vi "calcbuffers.vi"(3 "size":i32) -> (0 "wfsize":i32, 1 "# of frames":i32)   [LabVIEW 2015]
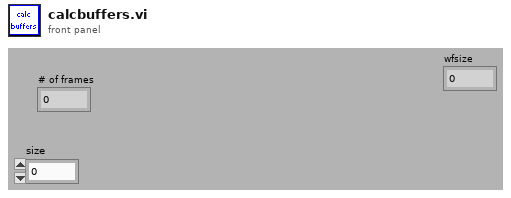
[diagram p1: front panel]
types:
  T1 = typedef "LVRectTypeDef.ctl" = cluster{"Left":i16, "Top":i16, "Right":i16, "Bottom":i16}
  T2 = cluster{"Xpixels":i32, "Vxminref":dbl, "Vxmaxref":dbl, "P":dbl, "Ypixels":i32, "Vyminref":dbl, "Vymaxref":dbl, "srate":sgl, "sAOxy":i32, "timeout":dbl, "type":string, "date":string, "time":string, "Colormap":u16, "Drawing Mode":u16, "Scanning Mode":u16, "square pixels":bool, "square matrix":bool, "Xpixels Img":i32, "Vx-min Img":dbl, "VX-max Img":dbl, "Ypixels Img":i32, "Vy-min Img":dbl, "Vy-max Img ":dbl, "Angle Img":dbl, "autoshutter":bool, "finite":bool, "cont":bool, "wavdet":bool, "measpoints":i32, "avpp":i32, "bufferAO":i32, "bufferAI":i32, "starttick":u32, "waveform":path, "Vx-ref":dbl, "Vy-ref":dbl, "refreshrate":dbl, "refreshbuffer":i32, "tt_cycles":i32, "motorref":refnum<k7>, "mirrorswitch":refnum<k7>, "sample mode":i32, "maxbufferAI":i32, "sampletreshold":dbl, "srateAODO":sgl, "bin":sgl, "Pel":sgl, "Angle draw":dbl, "srate Img":sgl, "ROIimg_plotbounds":T1, "auto OD":bool, "ODfilt":u16, "reset AO_DO":bool, "aAI":i32[], "aCI":i32[], "aAO":u32[], "aDO":u32[], "refwfsize":dbl}
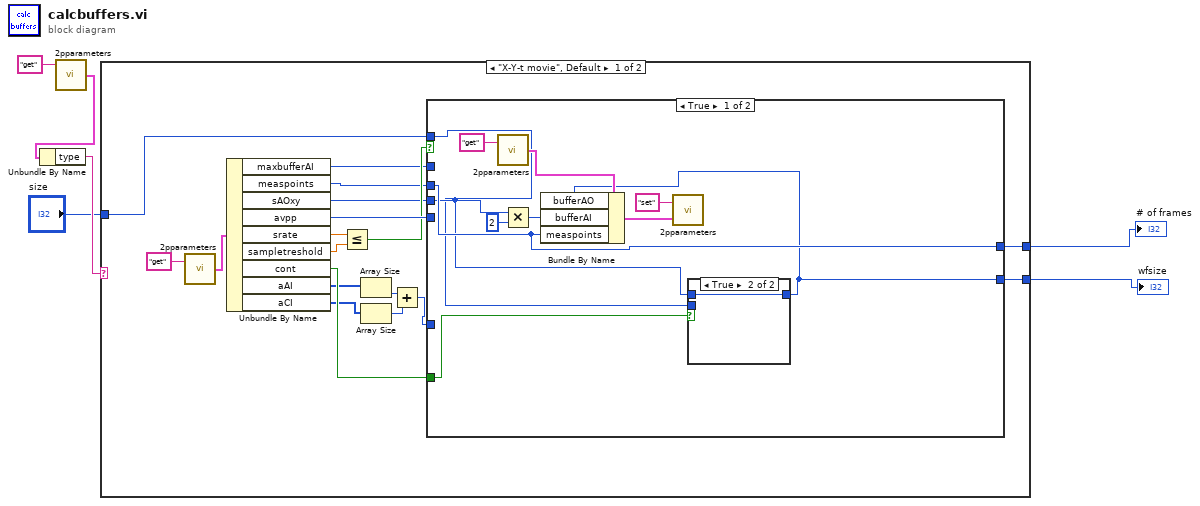
[diagram p0: block diagram]
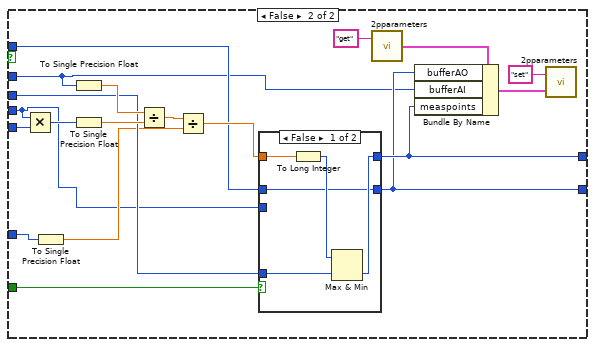
[diagram p3: hidden frame]
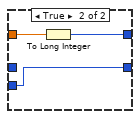
[diagram p4: hidden frame]
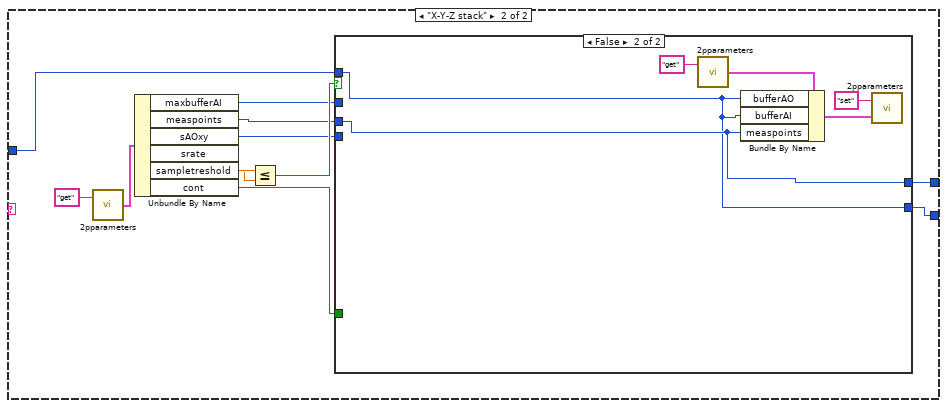
[diagram p5: hidden frame]
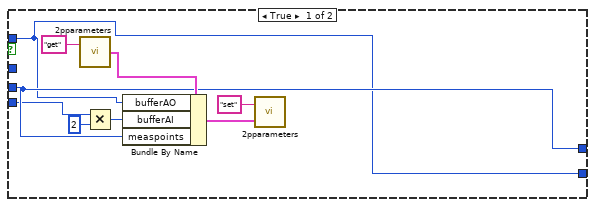
[diagram p6: hidden frame]
diagram:
  n1 = call "2pparameters.vi"("command"="get") -> ("params out"=w5:T2)  [unwired: 1 in]
  n2 = Unbundle By Name(w5) -> ("type"=w4:string)
  n3 = case shown="\"X-Y-t movie\", Default" w4 {
    tunnel: "size" -> [w9 w66]
    tunnel: [w8 w67] -> w2
    tunnel: [w7 w65] -> w1
    frame "X-Y-t movie", Default {
      n4 = call "2pparameters.vi"("command"="get") -> ("params out"=w23:T2)  [unwired: 1 in]
      n5 = Unbundle By Name(w23) -> ("maxbufferAI"=w16:i32, "measpoints"=w18:i32, "sAOxy"=w19:i32, "avpp"=w22:i32, "srate"=w21:sgl, "sampletreshold"=w17:dbl, "cont"=w15:bool, "aAI"=w14:i32[], "aCI"=w13:i32[])
      n6 = Less Or Equal?(x=w21, y=w17) -> (x <= y?=w20:bool)
      n7 = Array Size(array=w14) -> (size(s)=w12:i32)
      n8 = Array Size(array=w13) -> (size(s)=w11:i32)
      n9 = Add(x=w12, y=w11) -> (x+y=w10:i32)
      n10 = case shown="True" w20 {
        tunnel: w19 -> [w27 w40]
        tunnel: w22 -> [_ w52]
        tunnel: w10 -> [_ w47]
        tunnel: w18 -> [w29 w44]
        tunnel: w15 -> [w28 w45]
        tunnel: w16 -> [_ w38]
        tunnel: w9 -> [w26 w41]
        tunnel: [w29 w43] -> w8
        tunnel: [w25 w39] -> w7
        frame True {
          n11 = call "2pparameters.vi"("command"="get") -> ("params out"=w35:T2)  [unwired: 1 in]
          n12 = Multiply(x=w27, y=2) -> (x*y=w30:i32)
          n13 = case shown="True" w28 {
            tunnel: w27 -> [_ w37]
            tunnel: [w36 w37] -> w25
            tunnel: w26 -> [w36 _]
            frame False {
            }
            frame True {
            }
          }
          n14 = Bundle By Name(cluster=w35, "bufferAO"=w25, "bufferAI"=w30, "measpoints"=w29) -> (w34:T2)
          n15 = call "2pparameters.vi"("Params in"=w34, "command"="set") -> ()  [unwired: 1 out]
        }
        frame False {
          n16 = Multiply(x=w40, y=w52) -> (x*y=w51:i32)
          n17 = To Single Precision Float(number=w47) -> (single precision float=w42:sgl)
          n18 = To Single Precision Float(number=w38) -> (single precision float=w50:sgl)
          n19 = To Single Precision Float(number=w51) -> (single precision float=w49:sgl)
          n20 = Divide(x=w50, y=w49) -> (x/y=w48:sgl)
          n21 = Divide(x=w48, y=w42) -> (x/y=w46:sgl)
          n22 = case shown="False" w45 {
            tunnel: [w58 w64] -> w43
            tunnel: w46 -> [w61 w63]
            tunnel: w44 -> [w60 _]
            tunnel: [w57 w62] -> w39
            tunnel: w41 -> [w57 _]
            tunnel: w40 -> [_ w62]
            frame False {
              n23 = To Long Integer(number=w61) -> (32bit integer=w59:i32)
              n24 = Max & Min(x=w59, y=w60) -> (min(x,y)=w58:i32)  [unwired: 1 out]
            }
            frame True {
              n25 = To Long Integer(number=w63) -> (32bit integer=w64:i32)
            }
          }
          n26 = call "2pparameters.vi"("command"="get") -> ("params out"=w56:T2)  [unwired: 1 in]
          n27 = Bundle By Name(cluster=w56, "bufferAO"=w39, "bufferAI"=w38, "measpoints"=w43) -> (w55:T2)
          n28 = call "2pparameters.vi"("Params in"=w55, "command"="set") -> ()  [unwired: 1 out]
        }
      }
    }
    frame "X-Y-Z stack" {
      n29 = call "2pparameters.vi"("command"="get") -> ("params out"=w75:T2)  [unwired: 1 in]
      n30 = Unbundle By Name(w75) -> ("maxbufferAI"=w68:i32, "measpoints"=w71:i32, "sAOxy"=w72:i32, "srate"=w74:sgl, "sampletreshold"=w69:dbl, "cont"=w70:bool)
      n31 = Less Or Equal?(x=w74, y=w69) -> (x <= y?=w73:bool)
      n32 = case shown="False" w73 {
        tunnel: w72 -> [w78 _]
        tunnel: w71 -> [w79 w87]
        tunnel: w70 -> [_ _]
        tunnel: w68 -> [_ _]
        tunnel: [w79 w87] -> w67
        tunnel: w66 -> [w77 w86]
        tunnel: [w77 w86] -> w65
        frame True {
          n33 = call "2pparameters.vi"("command"="get") -> ("params out"=w85:T2)  [unwired: 1 in]
          n34 = Multiply(x=w78, y=2) -> (x*y=w80:i32)
          n35 = Bundle By Name(cluster=w85, "bufferAO"=w77, "bufferAI"=w80, "measpoints"=w79) -> (w84:T2)
          n36 = call "2pparameters.vi"("Params in"=w84, "command"="set") -> ()  [unwired: 1 out]
        }
        frame False {
          n37 = call "2pparameters.vi"("command"="get") -> ("params out"=w91:T2)  [unwired: 1 in]
          n38 = Bundle By Name(cluster=w91, "bufferAO"=w86, "bufferAI"=w86, "measpoints"=w87) -> (w90:T2)
          n39 = call "2pparameters.vi"("Params in"=w90, "command"="set") -> ()  [unwired: 1 out]
        }
      }
    }
  }
  "# of frames" <- w2
  "wfsize" <- w1
